vi "Filter Unexpired Paths.vi"(0 "Path Groups in":refnum<class "Path Group.lvclass">[](array[class]), 11 "error in":errorcluster) -> (4 "Path Groups out":refnum<class "Path Group.lvclass">[](array[class]), 6 "Path Count":i32, 10 "Paths Filtered out":refnum<class "Path.lvclass">[](array[class]), 15 "error out":errorcluster)   [LabVIEW 2023, in "RFFixtureCharact.Public.lvlib"]
uses:
  RFFixtureCharact.Public.lvlib
  Common/Base Classes/Path Group/Path Group.lvclass
  Common/Base Classes/Path/Path.lvclass
  Common/RFCalAndFixtureCharact.Common.lvlib
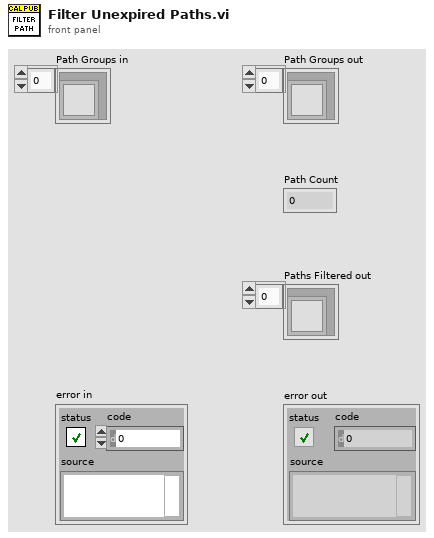
[diagram p1: front panel]
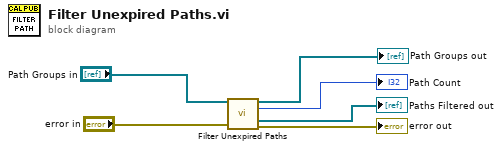
[diagram p0: block diagram]
diagram:
  n1 = call "Filter Unexpired Paths.vi"("Path Groups in"="Path Groups in", "Error in (no error)"="error in") -> ("Path Groups out"=→"Path Groups out":refnum<class "Path Group.lvclass">[], "Path Count"=→"Path Count":i32, "Paths Filtered out"=→"Paths Filtered out":refnum<class "Path.lvclass">[], "Error out"=→"error out":errorcluster)  [unwired: 10 in]
